vi "PXI4072 Get Instrument Status .vi"(8 "error in (no error)":errorcluster, 11 "Instrument Status":T1) -> (0 "error out":errorcluster, 2 "selected enum name":string, 3 "enum names":string[](array[string]))   [LabVIEW 2026]
uses:
  <vilib>/Utility/Data Type/NI_Data Type.lvlib
  App Types/Enums/PXI4072 Instrument Status.ctl
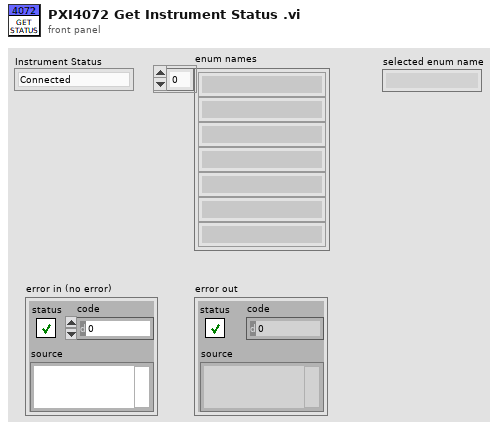
[diagram p1: front panel]
types:
  T1 = typedef "PXI4072 Instrument Status.ctl" = enum16{"Connected", "Ready", "Disconnected"}
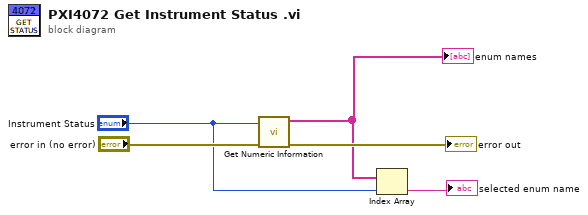
[diagram p0: block diagram]
diagram:
  n1 = call <vilib>:"Get Numeric Information.vi"("error in (no error)"="error in (no error)", "variant"="Instrument Status") -> ("error out"=→"error out":errorcluster, "enum names"=w3:string[])  [unwired: 6 in, 2 out]
  "enum names" <- w3
  n2 = Index Array(array=w3, index="Instrument Status") -> (element=→"selected enum name":string)
